vi "APC_9049_HRL_ZeroPhaseFIlterBP.vi"(2 "Init value removal":bool, 3 "IIR Filter Cluster":T1, 4 "Pcyl":dbl[](array[numeric])) -> (0 "Pcylfilt":dbl[](array[numeric]), 1 "Pressure filtering":dbl[][](graph))   [LabVIEW 2020]
uses:
  <vilib>/Analysis/3filter.llb/Zero Phase Filter (Cascade, DBL).vi
  <vilib>/Analysis/NI_AALBase.lvlib
panel:
  in  "Graph":bool
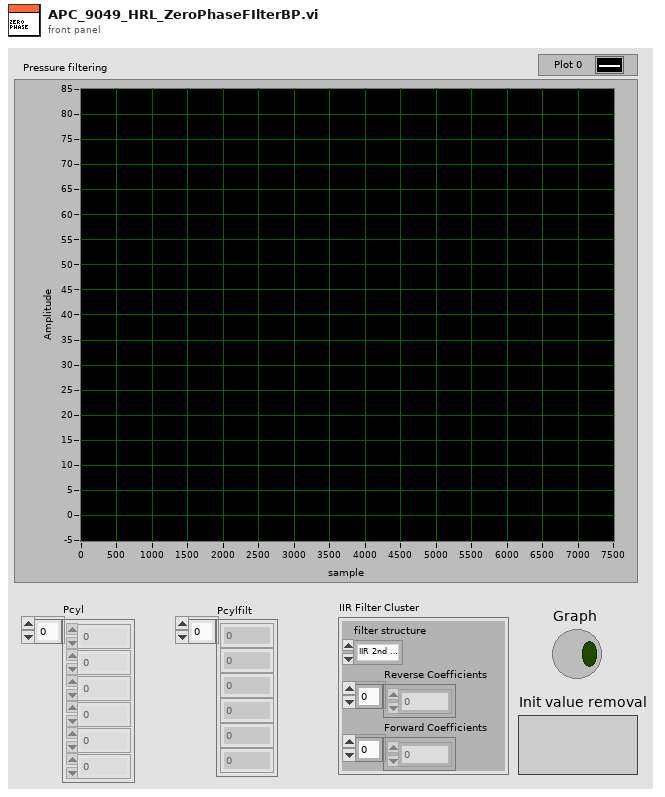
[diagram p1: front panel]
types:
  T1 = cluster{"filter structure":enum32{"IIR 2nd Order", "IIR 4th Order"}, "Reverse Coefficients":dbl[], "Forward Coefficients":dbl[]}
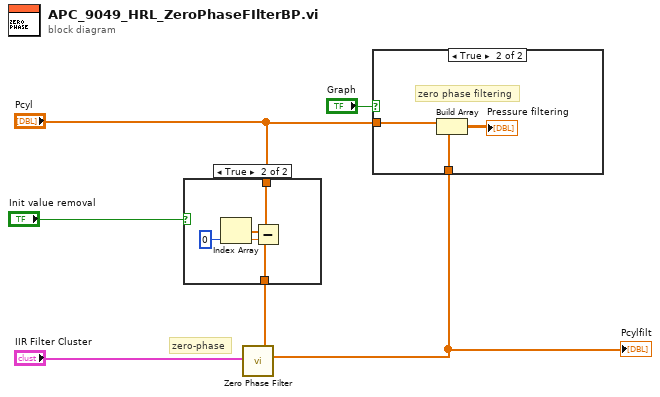
[diagram p0: block diagram]
diagram:
  # "zero-phase"
  n1 = case shown="True" "Init value removal" {
    tunnel: "Pcyl" -> [w7 w11]
    tunnel: [w7 w10] -> w5
    frame False {
    }
    frame True {
      n2 = Index Array(array=w11, index=0) -> (element=w9:dbl)
      n3 = Subtract(x=w11, y=w9) -> (x-y=w10:dbl[])
    }
  }
  n4 = call-poly <vilib>:"Zero Phase Filter.vi"("IIR Filter Cluster"="IIR Filter Cluster", "X"=w5) -> ("Filtered X"=w1:dbl[])  [unwired: 8 in, 1 out]
  "Pcylfilt" <- w1
  n5 = case shown="True" "Graph" {
    tunnel: "Pcyl" -> [_ w14]
    tunnel: w1 -> [_ w13]
    frame False {
    }
    frame True {
      # "zero phase filtering"
      n6 = Build Array(w14, w13) -> (→"Pressure filtering":dbl[][])
    }
  }
